vi "Get Active Tag.vi"(8 "error in (no error)":errorcluster, 11 "Tree_LVOOP in":refnum<class "Tree Class.lvclass">) -> (0 "error out":errorcluster, 2 "Active Tag":refnum<class "Tree Tag Class.lvclass">, 3 "Tree_LVOOP out":refnum<class "Tree Class.lvclass">)   [LabVIEW 2012, in "Tree Tools.lvlib" / "Tree Class.lvclass"]
uses:
  Tree Class.lvclass
  Tree Tag Class/Tree Tag Class.lvclass
  Tree Class.lvclass/Tree Class.ctl
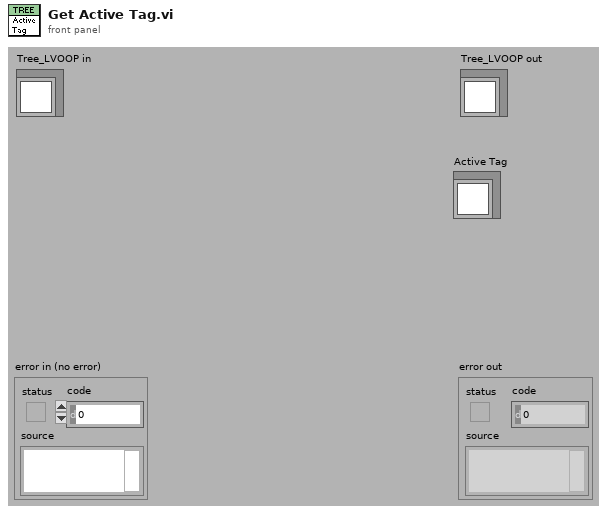
[diagram p1: front panel]
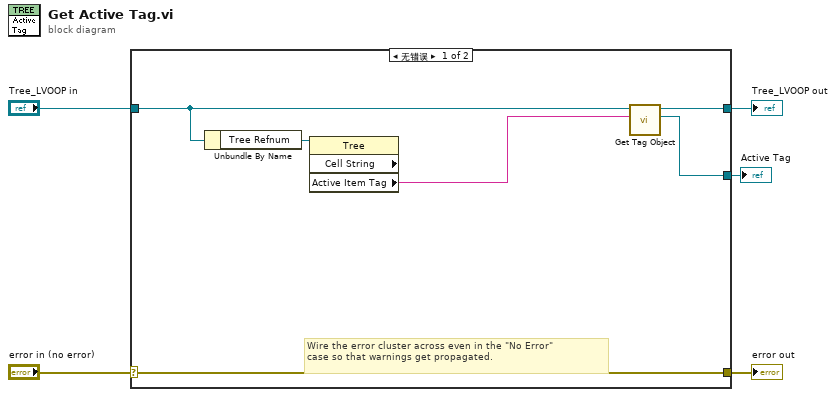
[diagram p0: block diagram]
diagram:
  n1 = case shown="无错误" "error in (no error)" {
    selector: "error in (no error)" -> [w11 w13]
    tunnel: [w11 w13] -> w4
    tunnel: [w8 w12] -> w2
    tunnel: "Tree_LVOOP in" -> [w9 w12]
    tunnel: [w6 _] -> w1
    frame No Error {
      # "Wire the error cluster across even in the \"No Error\"\ncase so that warnings get propagated."
      n2 = Unbundle By Name(w9) -> ("Tree Refnum"=w10:refnum<vi>)
      n3 = property class="Tree" props=["Cell String", "Active Item Tag"](reference=w10) -> ("Active Item Tag"=w7:string)  [unwired: 1 in, 3 out]
      n4 = call-dynamic "Get Tag Object.vi"("Tag (string)"=w7, "Tree_LVOOP in"=w9) -> ("Tag"=w6:refnum<class "Tree Tag Class.lvclass">, "Tree_LVOOP out"=w8:refnum<class "Tree Class.lvclass">)  [unwired: 2 in, 6 out]
    }
    frame Error {
    }
  }
  "error out" <- w4
  "Tree_LVOOP out" <- w2
  "Active Tag" <- w1
